vi "labview_2.vi"() -> ()   [LabVIEW 2025]
panel:
  in  "Patient":T1
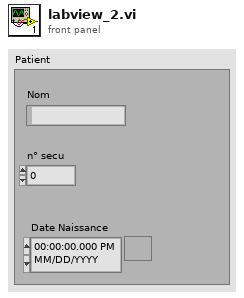
[diagram p1: front panel]
types:
  T1 = cluster{"Nom":string, "n° secu\n":dbl, "Date Naissance":timestamp}
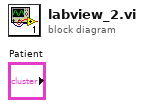
[diagram p0: block diagram]
diagram:
